vi "Laser Config.vi"(8 "error in (no error)":errorcluster, 9 "Gain":u16, 10 "Init Power":u16, 11 "Select Probe":i32) -> (0 "error out":errorcluster)   [LabVIEW 2015, in "Tool Interface.lvlib"]
uses:
  Tool Interface.lvlib
  Tool Typedefs/_Laser Params Cluster--typedef.ctl
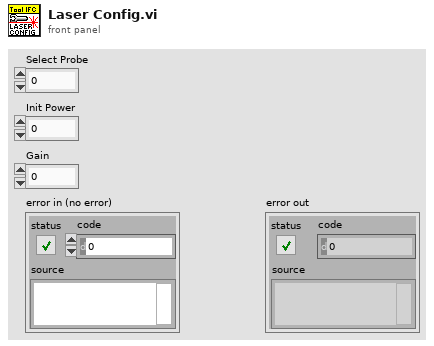
[diagram p1: front panel]
types:
  T1 = typedef "_Laser Params Cluster--typedef.ctl" = cluster{"Mode":i16, "Gain":u16, "Init":u16}
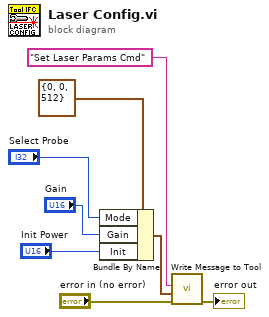
[diagram p0: block diagram]
diagram:
  n1 = Bundle By Name(cluster=T1 {"Mode"=0, "Gain"=0, "Init"=512} ("_Laser Params Cluster--typedef"), "Mode"="Select Probe", "Gain"="Gain", "Init"="Init Power") -> (w3:T1)
  n2 = call "Write Message to Tool.vi"("error in (no error)"="error in (no error)", "Message Data"=w3, "Message"="Set Laser Params Cmd") -> ("error out"=→"error out":errorcluster)  [unwired: 8 in]
